vi "SignalsSimulator.vi"() -> ()   [LabVIEW 2011]
uses:
  <vilib>/measure/NI_MABase.lvlib
panel:
  in  "?":bool
  out "error out 0":errorcluster
  out "error out 1":errorcluster
  in  "Sampling2":cluster{"Fs":dbl, "#s":dbl}={"Fs"=1000.0, "#s"=1000.0} {"#s" format="%_6g"; "Fs" format="%_6g"}
  in  "Sampling1":cluster{"Fs":dbl, "#s":dbl}={"Fs"=1000.0, "#s"=1000.0} {"#s" format="%_6g"; "Fs" format="%_6g"}
  out "Waveform Graph":waveform(dbl)[](graph)
  in  "Reset phase2":bool
  in  "Reset phase1":bool
  in  "Phase2":dbl
  in  "Phase1":dbl
  in  "Frequency2":dbl=2.0
  in  "Frequency1":dbl=2.0
  in  "Amplitude2":dbl=2.0
  in  "Amplitude 1":dbl=4.0
  # "334AB ALEXANDRESCU Anda\nGenerarea si afisarea simultana a doua semnale"
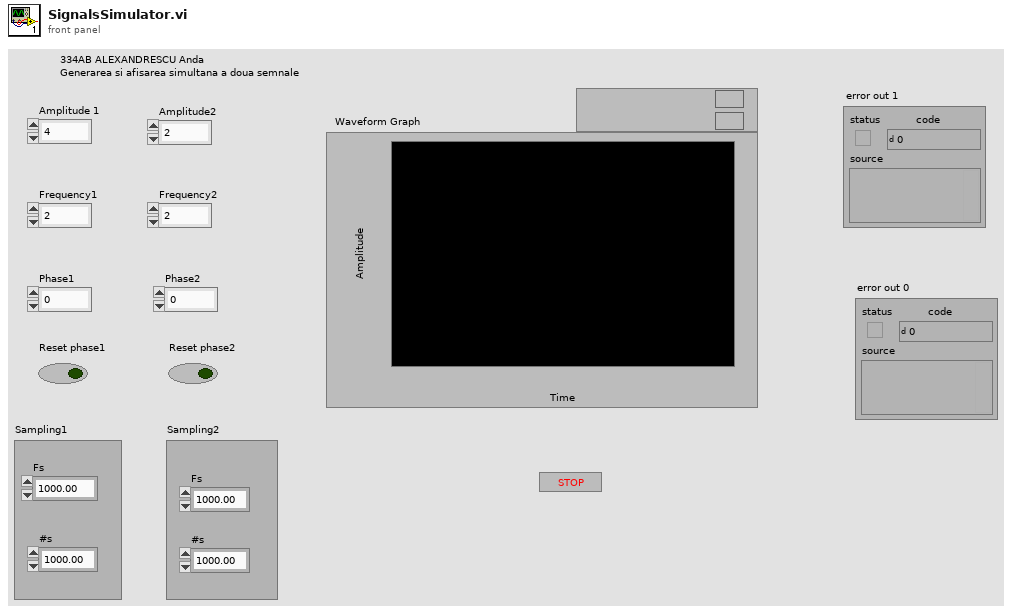
[diagram p1: front panel]
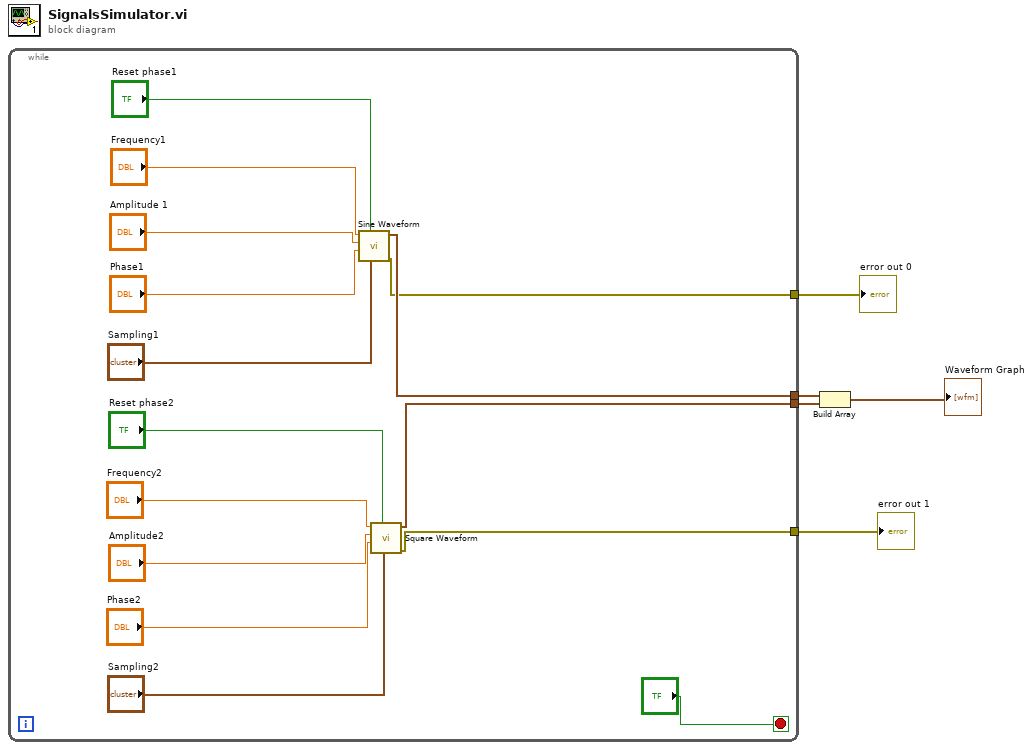
[diagram p0: block diagram]
diagram:
  n1 = while {
    tunnel: [w9] -> w5
    tunnel: [w8] -> w4
    tunnel: [w7] -> w3
    tunnel: [w6] -> w2
    stop <- "?" stop-if-true
    n2 = call <vilib>:"Sine Waveform.vi"("sampling info"="Sampling1", "reset signal"="Reset phase1", "phase"="Phase1", "amplitude"="Amplitude 1", "frequency"="Frequency1") -> ("error out"=w6:errorcluster, "signal out"=w9:waveform(dbl))  [unwired: 5 in]
    n3 = call <vilib>:"Square Waveform.vi"("sampling info"="Sampling2", "reset signal"="Reset phase2", "phase"="Phase2", "amplitude"="Amplitude2", "frequency"="Frequency2") -> ("error out"=w7:errorcluster, "signal out"=w8:waveform(dbl))  [unwired: 5 in]
  }
  "error out 1" <- w3
  "error out 0" <- w2
  n4 = Build Array(w5, w4) -> (→"Waveform Graph":waveform(dbl)[])
